vi "demoUI_2.vi"() -> ()   [LabVIEW 2013]
uses:
  Controls/Status TYP.ctl
  Controls/State TYP.ctl
panel:
  in  "Status":T1
  in  "Teacher":bool
  in  "Setup":bool
  in  "Experiment":bool
  out "MainTab":T2(tab)
  out "SetupTab":enum32{"Page 4", "Page 1", "Page 2", "Page 3"}(tab)
  out "Step #":i32
  in  "Setup Next":bool
  in  "Setup Previous":bool
  in  "Log Save":bool
  in  "Log Stop":bool
  in  "Log Start":bool
  out "Numeric 2":dbl format="%.1f"
  out "Color Ramp 2":dbl(ramp)
  out "Numeric":dbl format="%.1f"
  out "Waveform Chart 2":cluster{"Slide":dbl, "One Cube":dbl}(graph)
  out "Color Ramp":dbl(ramp)
  # "Welcome!"
  # "Press these buttons\nto get started"
  # "Setup"
  # "Welcome to the PLTW myDAQ Experiment!\n\nIn this experiment, you will learn about temperature\nand how different events affect temperature.\n\nYou will use the NI myDAQ to perform this experiment.\n\nClick the 'Next' button at the bottom to go to the next step"
  # "First, find your myDAQ"
  # "Plug the myDAQ into the computer with a USB cable"
  # "Place one ice Cube in one cup\nand two ice cubes in another cup"
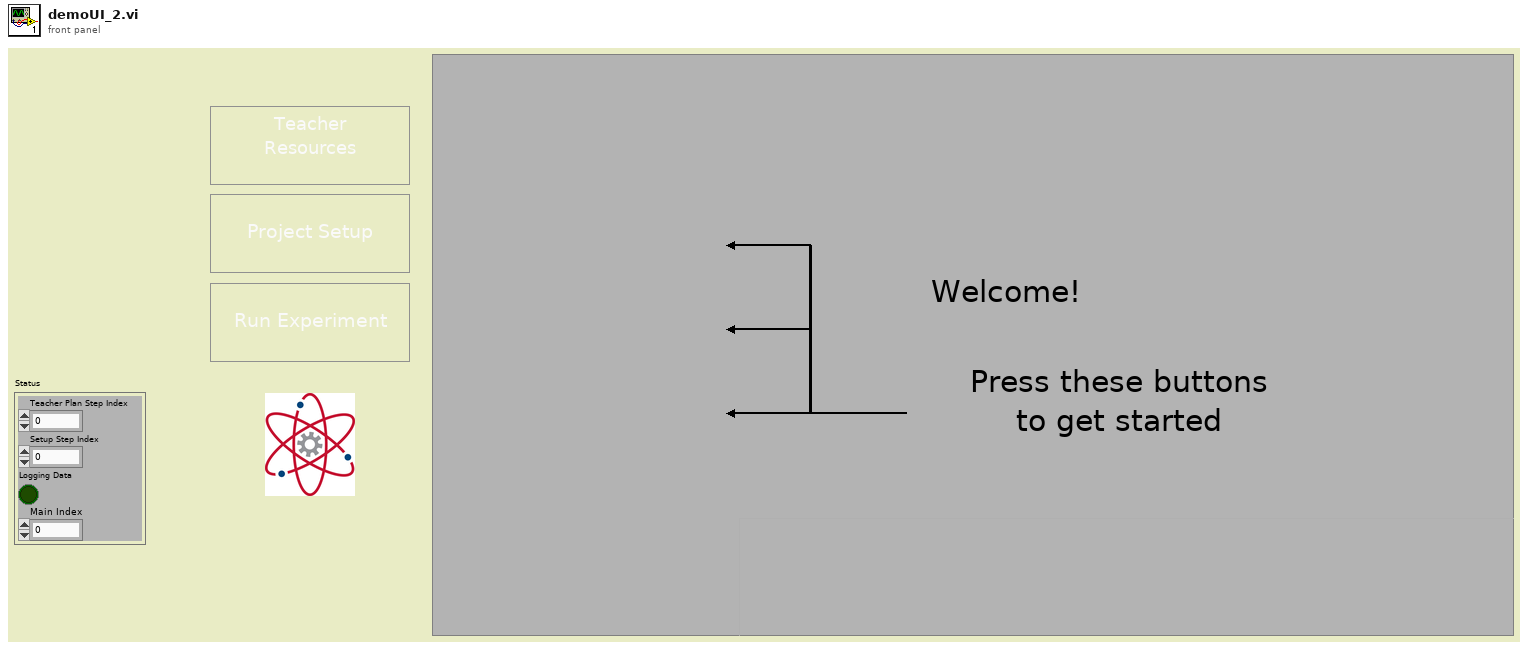
[diagram p1: front panel]
types:
  T1 = typedef "Status TYP.ctl" = cluster{"Teacher Plan Step Index":i32, "Setup Step Index":i32, "Logging Data":bool, "Main Index":i32}
  T2 = enum32{"Welcome", "Teacher Lesson Plan", "Project Setup", "Experiment"}
  T3 = typedef "State TYP.ctl" = enum16{"Idle", "Init", "Exit", "<-- Tabs -->", "Teacher", "Setup", "Experiment", "<-- Actions -->", "Setup Next", "Setup Previous", "Teacher Next", "Teacher Previous", "Log Start", "Log Stop", "Log Save", "UI Update"}
  T4 = enum8{"Enabled", "Disabled", "Disabled and Grayed Out"}
  T5 = enum32{"invalid app kind", "Development System", "Run Time System", "Student Edition", "Embedded LabVIEW", "Evaluation", "Custom"}
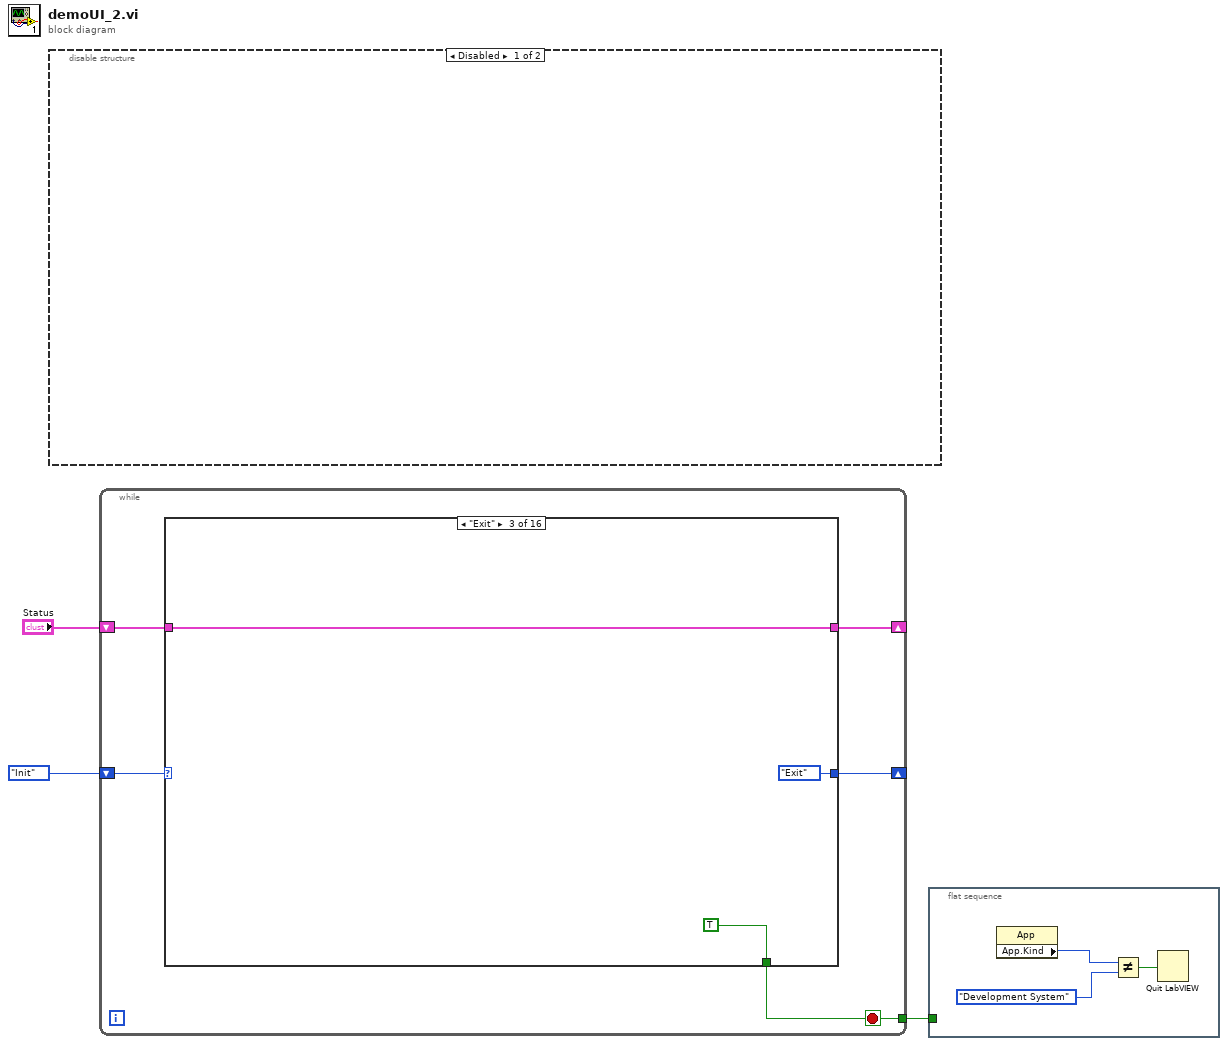
[diagram p0: block diagram]
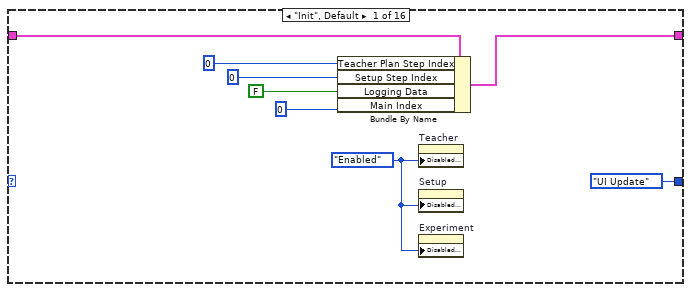
[diagram p3: hidden frame]
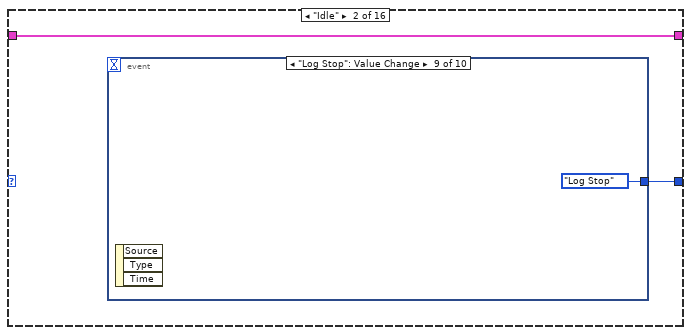
[diagram p4: hidden frame]
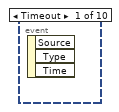
[diagram p5: hidden frame]
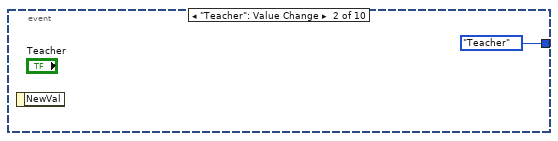
[diagram p6: hidden frame]
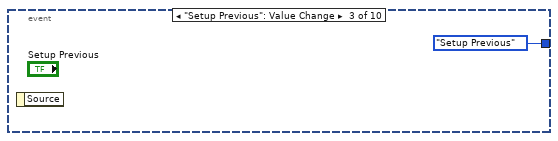
[diagram p7: hidden frame]
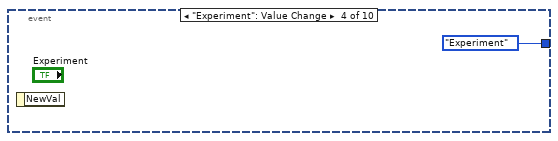
[diagram p8: hidden frame]
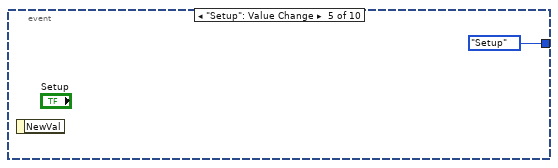
[diagram p9: hidden frame]
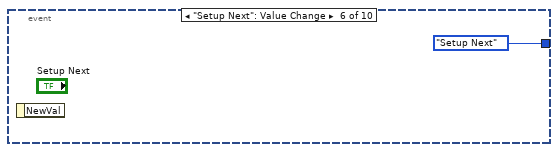
[diagram p10: hidden frame]
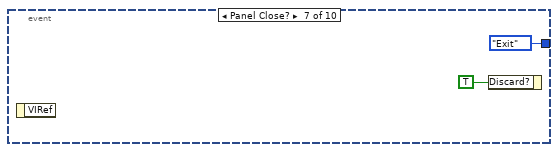
[diagram p11: hidden frame]
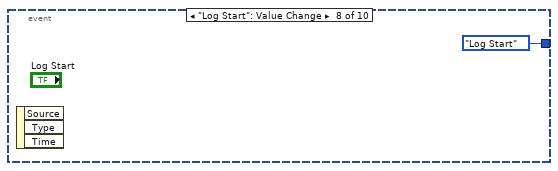
[diagram p12: hidden frame]
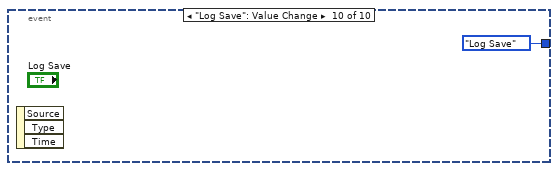
[diagram p13: hidden frame]
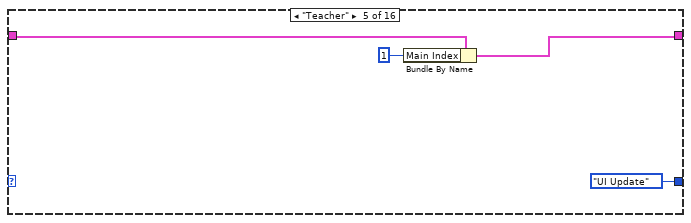
[diagram p15: hidden frame]
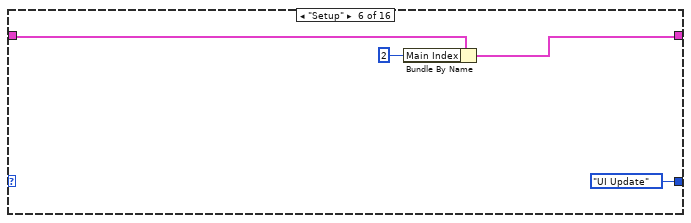
[diagram p16: hidden frame]
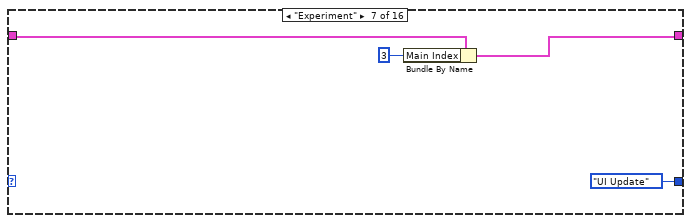
[diagram p17: hidden frame]
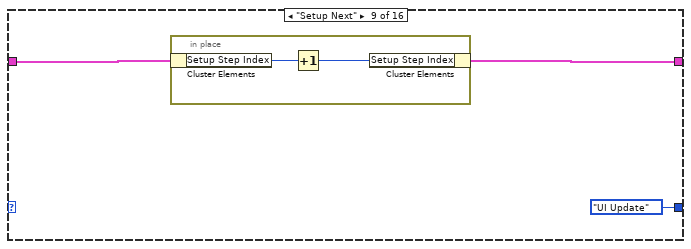
[diagram p19: hidden frame]
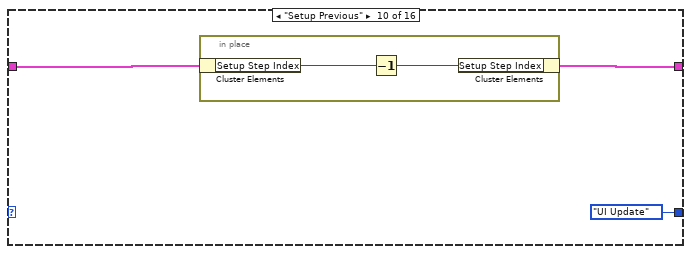
[diagram p20: hidden frame]
diagram:
  n1 = disable-structure shown="Disabled" {
    frame Disabled {
    }
    frame Enabled {
    }
  }
  n2 = while {
    shift-right: [w7] -> _
    shift-left: State_TYP."Init" -> [w8]
    shift-right: [w5] -> _
    shift-left: "Status" -> [w6]
    tunnel: [w4] -> w1
    stop <- w4 stop-if-true
    n3 = case shown="\"Exit\"" w8 {
      tunnel: [State_TYP."UI Update" w18 State_TYP."Exit" _ State_TYP."UI Update" State_TYP."UI Update" State_TYP."UI Update" _ State_TYP."UI Update" State_TYP."UI Update" State_TYP."UI Update" State_TYP."UI Update" _ State_TYP."Log Stop" State_TYP."UI Update" _] -> w7
      tunnel: w6 -> [w16 w17 w31 w32 w35 w39 w43 w45 w47 w53 w58 w63 w69 w76 w84 w85]
      tunnel: [w15 w17 w31 w32 w34 w38 w42 w45 w46 w51 w57 w62 w69 w76 w84 w85] -> w5
      tunnel: [_ _ TRUE _ _ _ _ _ _ _ _ _ _ _ _ _] -> w4
      frame "Init", Default {
        w9 = T4."Enabled" ("Disabled")
        n4 = Bundle By Name(cluster=w16, "Teacher Plan Step Index"=0, "Setup Step Index"=0, "Logging Data"=FALSE, "Main Index"=0) -> (w15:T1)
        n5 = property on="Teacher" class="Bool"("DisabledEnum"=w9) -> ()  [unwired: 2 in, 2 out]
        n6 = property on="Setup" class="Bool"("DisabledEnum"=w9) -> ()  [unwired: 2 in, 2 out]
        n7 = property on="Experiment" class="Bool"("DisabledEnum"=w9) -> ()  [unwired: 2 in, 2 out]
      }
      frame "Idle" {
        n8 = event shown="[8] \"Log Stop\": Value Change" {
          selector: _ -> [_ _ _ _ _ _ _ _ _ _]
          dyn-events: _ -> [_ _ _ _ _ _ _ _ _ _]
          timeout: _ -> [_ _ _ _ _ _ _ _ _ _]
          tunnel: [_ State_TYP."Teacher" State_TYP."Setup Previous" State_TYP."Experiment" State_TYP."Setup" State_TYP."Setup Next" State_TYP."Exit" State_TYP."Log Start" State_TYP."Log Stop" State_TYP."Log Save"] -> w18
          event Timeout {
            n9 = event-data() -> ()  [unwired: 1 in, 3 out]
          }
          event "Teacher": Value Change {
            n10 = event-data() -> ()  [unwired: 1 in, 1 out]
          }
          event "Setup Previous": Value Change {
            n11 = event-data() -> ()  [unwired: 1 in, 1 out]
          }
          event "Experiment": Value Change {
            n12 = event-data() -> ()  [unwired: 1 in, 1 out]
          }
          event "Setup": Value Change {
            n13 = event-data() -> ()  [unwired: 1 in, 1 out]
          }
          event "Setup Next": Value Change {
            n14 = event-data() -> ()  [unwired: 1 in, 1 out]
          }
          event Panel Close? {
            n15 = event-data() -> ()  [unwired: 1 in, 1 out]
            n16 = event-data("Discard?"=TRUE) -> ()  [unwired: 1 in, 1 out]
          }
          event "Log Start": Value Change {
            n17 = event-data() -> ()  [unwired: 1 in, 3 out]
          }
          event "Log Stop": Value Change {
            n18 = event-data() -> ()  [unwired: 1 in, 3 out]
          }
          event "Log Save": Value Change {
            n19 = event-data() -> ()  [unwired: 1 in, 3 out]
          }
        }
      }
      frame "Exit" {
      }
      frame "<-- Tabs -->" {
      }
      frame "Teacher" {
        n20 = Bundle By Name(cluster=w35, "Main Index"=1) -> (w34:T1)
      }
      frame "Setup" {
        n21 = Bundle By Name(cluster=w39, "Main Index"=2) -> (w38:T1)
      }
      frame "Experiment" {
        n22 = Bundle By Name(cluster=w43, "Main Index"=3) -> (w42:T1)
      }
      frame "<-- Actions -->" {
      }
      frame "Setup Next" {
        n23 = in-place {
          n24 = in-place-cluster #1(w47) -> ("Setup Step Index"=w50:i32)
          n25 = Increment(x=w50) -> (x+1=w49:i32)
          n26 = in-place-cluster #1("Setup Step Index"=w49) -> (w46:T1)
        }
      }
      frame "Setup Previous" {
        n27 = in-place {
          n28 = in-place-cluster #2(w53) -> ("Setup Step Index"=w55:i32)
          n29 = Decrement(x=w55) -> (x-1=w54:i32)
          n30 = in-place-cluster #2("Setup Step Index"=w54) -> (w51:T1)
        }
      }
      frame "Teacher Next" {
        n31 = in-place {
          n32 = in-place-cluster #3(w58) -> ("Teacher Plan Step Index"=w60:i32)
          n33 = Increment(x=w60) -> (x+1=w59:i32)
          n34 = in-place-cluster #3("Teacher Plan Step Index"=w59) -> (w57:T1)
        }
      }
      frame "Teacher Previous" {
        n35 = in-place {
          n36 = in-place-cluster #4(w63) -> ("Teacher Plan Step Index"=w65:i32)
          n37 = Decrement(x=w65) -> (x-1=w64:i32)
          n38 = in-place-cluster #4("Teacher Plan Step Index"=w64) -> (w62:T1)
        }
      }
      frame "UI Update" {
        n39 = Unbundle By Name(w69) -> ("Setup Step Index"=w68:i32, "Main Index"=→"MainTab":i32)
        "SetupTab" <- w68
        n40 = Increment(x=w68) -> (x+1=→"Step #":i32)
      }
      frame "Log Start" {
        w72 = T4."Disabled and Grayed Out" ("Disabled")
        w74 = dbl[] [76.0, 76.0, 76.0, 76.0, 76.0, 76.0, 76.0, 75.3529411764706, 74.49019607843138, 73.62745098039215, 72.76470588235294, 71.90196078431373, 71.03921568627452, 69.31372549019608, 68.01960784313725, 66.50980392156863, 64.7843137254902, 63.70588235294118, 62.411764705882355, 61.76470588235294, 60.90196078431373, 60.254901960784316, 59.1764705882353, 58.09803921568628, 57.01960784313726, 55.72549019607843, 54.431372549019606, 53.35294117647059, 52.05882352941177, 51.19607843137255, 50.549019607843135, 49.470588235294116, 48.6078431372549, 47.745098039215684, 46.88235294117647, 46.23529411764706, 45.588235294117645, 44.294117647058826, 43.431372549019606, 42.78431372549019, 41.490196078431374, 40.411764705882355, 39.333333333333336, 38.68627450980392, 38.254901960784316, 37.8235294117647, 37.1764705882353, 36.745098039215684, 36.529411764705884, 36.31372549019608, 35.666666666666664, 35.450980392156865, 34.80392156862745, 34.372549019607845, 34.372549019607845, 34.372549019607845, 34.15686274509804, 34.15686274509804, 34.15686274509804, 34.15686274509804, 34.15686274509804, 33.94117647058823, 33.94117647058823, 33.509803921568626, 33.509803921568626, 33.294117647058826, 33.07843137254902, 33.07843137254902, 32.86274509803921, 32.64705882352941, 32.64705882352941, 32.431372549019606, 32.431372549019606, 32.21568627450981, 32.21568627450981, 32.0, 32.0, 32.0, 32.0, 32.0, 32.0, 32.0, 32.0, 32.0, 32.0, 32.0, 32.0, 32.0, 32.0, 32.0, 32.0, 32.0, 32.0, 32.0, 32.0, 32.0, 32.0, 32.0, 32.0, 32.0, 32.0, 32.0, 32.0, 32.0, 32.0, 32.0, 32.0, 32.0, 32.0]  # two cubes
        w73 = dbl[] [76.0, 76.0, 76.0, 76.0, 76.0, 76.0, 76.0, 76.0, 76.0, 76.0, 76.0, 75.45679012345678, 75.45679012345678, 74.64197530864197, 73.82716049382717, 73.28395061728395, 72.74074074074073, 72.74074074074073, 72.74074074074073, 72.46913580246914, 71.92592592592592, 71.38271604938271, 70.8395061728395, 70.29629629629629, 70.02469135802468, 69.20987654320987, 68.39506172839506, 67.30864197530865, 66.76543209876543, 66.22222222222221, 65.67901234567901, 64.86419753086419, 63.77777777777778, 62.96296296296296, 62.148148148148145, 61.33333333333333, 60.24691358024691, 59.7037037037037, 59.432098765432094, 58.34567901234568, 57.25925925925926, 56.98765432098765, 55.901234567901234, 55.08641975308642, 54.0, 52.641975308641975, 51.82716049382716, 51.28395061728395, 50.19753086419753, 49.65432098765432, 48.839506172839506, 48.5679012345679, 47.48148148148148, 46.39506172839506, 45.58024691358025, 44.76543209876543, 43.95061728395061, 42.864197530864196, 42.32098765432099, 42.32098765432099, 42.32098765432099, 41.50617283950617, 41.50617283950617, 40.96296296296296, 40.96296296296296, 40.41975308641975, 40.41975308641975, 40.148148148148145, 39.876543209876544, 39.876543209876544, 39.876543209876544, 39.876543209876544, 39.876543209876544, 39.876543209876544, 39.876543209876544, 39.333333333333336, 39.333333333333336, 39.06172839506173, 39.06172839506173, 38.79012345679012, 38.51851851851852, 37.7037037037037, 37.4320987654321, 37.4320987654321, 37.160493827160494, 36.888888888888886, 36.888888888888886, 36.34567901234568, 36.074074074074076, 35.80246913580247, 35.53086419753087, 35.53086419753087, 34.98765432098765, 34.44444444444444, 34.44444444444444, 34.17283950617284, 33.629629629629626, 33.358024691358025, 33.08641975308642, 32.81481481481482, 32.54320987654321, 32.27160493827161, 32.0, 32.0, 32.0, 32.0, 32.0, 32.0, 32.0, 32.0, 32.0, 32.0, 32.0, 32.0, 32.0, 32.0, 32.0, 32.0, 32.0, 32.0, 32.0, 32.0, 32.0, 32.0, 32.0]  # one cube
        n41 = property on="Teacher" class="Bool"("DisabledEnum"=w72) -> ()  [unwired: 2 in, 2 out]
        n42 = property on="Setup" class="Bool"("DisabledEnum"=w72) -> ()  [unwired: 2 in, 2 out]
        n43 = property on="Experiment" class="Bool"("DisabledEnum"=w72) -> ()  [unwired: 2 in, 2 out]
        n44 = property on="Waveform Chart 2" class="WFChart (strict)"("History Data"=cluster{"Slide":dbl, "One Cube":dbl}[] []) -> (error out=w71:errorcluster)  [unwired: 2 in, 1 out]
        n45 = for {
          tunnel: w73 -> [w78] mode=indexing
          tunnel: w74 -> [w79] mode=indexing
          tunnel: w71 -> [_]
          stop <- "Log Stop" stop-if-true
          n46 = Bundle("Slide"=w79, "One Cube"=w78) -> (→"Waveform Chart 2":cluster{"Slide":dbl, "One Cube":dbl})  [unwired: 1 in]
          n47 = Wait (ms)(milliseconds to wait=u32 256) -> ()  [unwired: 1 out]
          "Color Ramp" <- w78
          "Color Ramp 2" <- w79
          "Numeric 2" <- w79
          "Numeric" <- w78
        }
      }
      frame "Log Stop" {
        w83 = T4."Enabled" ("Disabled")
        n48 = property on="Teacher" class="Bool"("DisabledEnum"=w83) -> ()  [unwired: 2 in, 2 out]
        n49 = property on="Setup" class="Bool"("DisabledEnum"=w83) -> ()  [unwired: 2 in, 2 out]
        n50 = property on="Experiment" class="Bool"("DisabledEnum"=w83) -> ()  [unwired: 2 in, 2 out]
      }
      frame "Log Save" {
      }
    }
  }
  n51 = flat-sequence {
    tunnel: w1 -> [_]
    frame #0 {
      n52 = property class="App"() -> ("App.Kind"=w88:T5)  [unwired: 2 in, 2 out]
      n53 = Not Equal?(x=w88, y=T5."Development System" ("Application:Kind")) -> (x != y?=w86:bool)
      n54 = Quit LabVIEW(quit? (T)=w86) -> ()
    }
  }
